vi "ABB Run Up report.vi"(10 "Report in":string) -> (2 "Report out":string)   [LabVIEW 2017]
uses:
  ABB global.vi
panel:
  out "Run Up Speed":T1(graph)
  out "Run Up Current":T1(graph)
  out "Run Up Voltage":T1(graph)
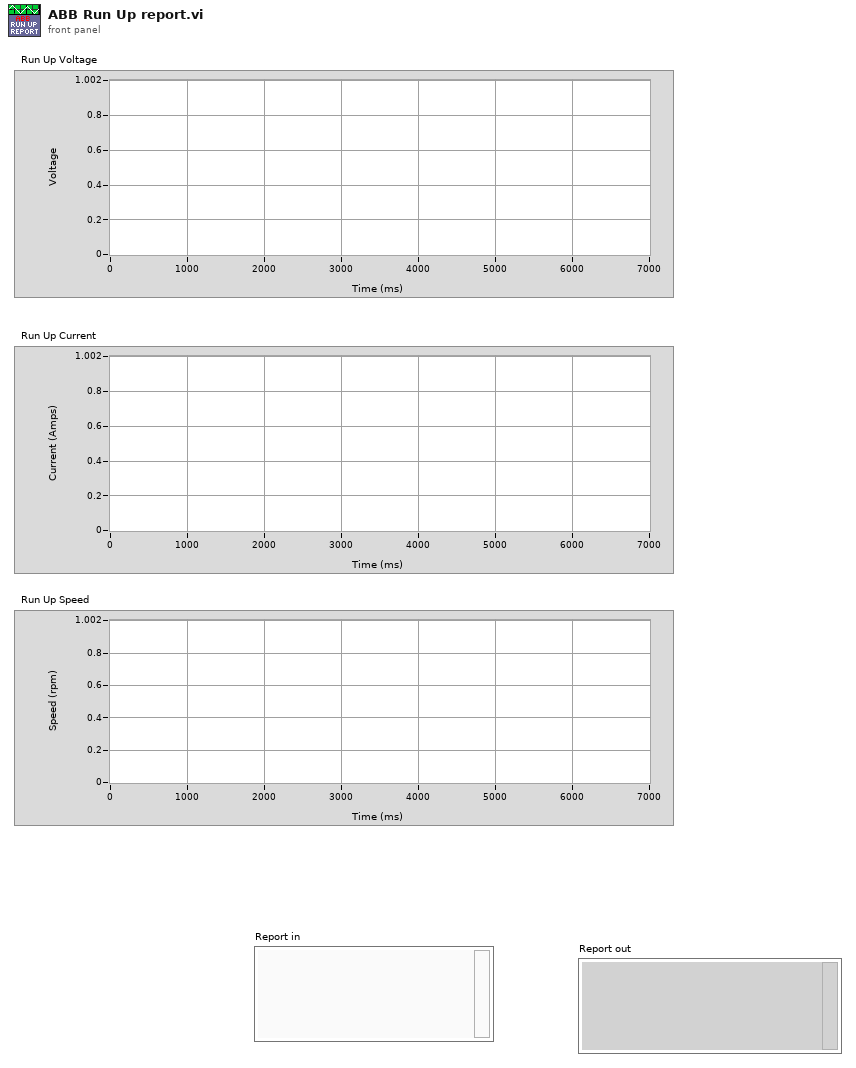
[diagram p1: front panel]
types:
  T1 = cluster{"No load test results":dbl[], "No load test results":dbl[]}
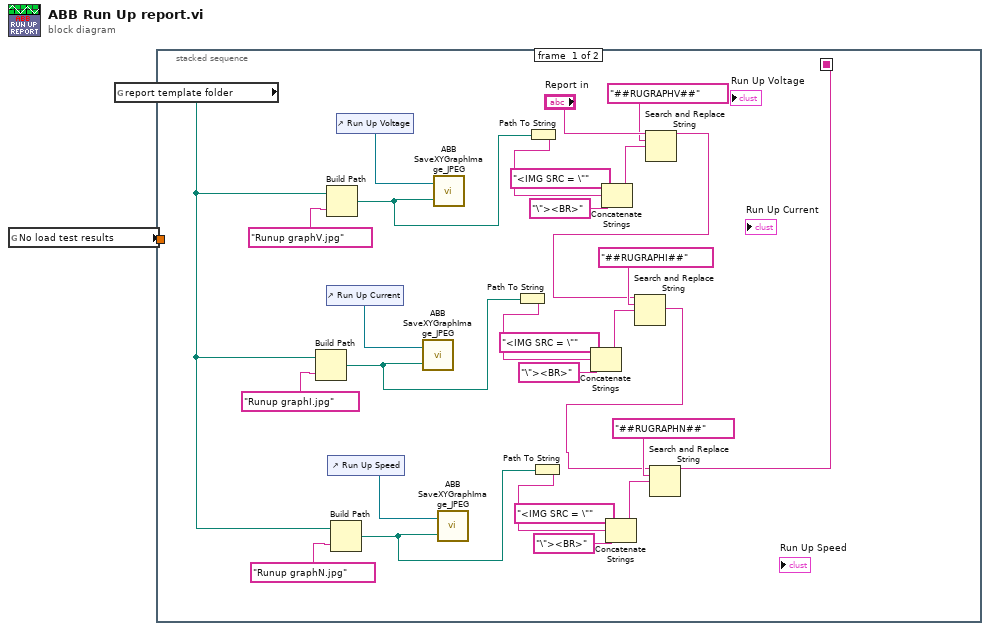
[diagram p0: block diagram]
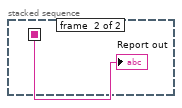
[diagram p2: hidden frame]
diagram:
  n1 = global read "ABB global.vi" "No load test results"() -> (w1:dbl[][])
  n2 = stacked-sequence {
    seq-local: [w2 _] -> [_ w31]
    tunnel: w1 -> [_ _]
    frame #0 {
      n3 = global read "ABB global.vi" "report template folder"() -> (w7:path)
      n4 = Build Path(base path=w7, name or relative path="Runup graphI.jpg") -> (appended path=w18:path)
      n5 = Build Path(base path=w7, name or relative path="Runup graphV.jpg") -> (appended path=w26:path)
      n6 = control-ref of="Run Up Current"() -> (w6:refnum<vi>)
      n7 = control-ref of="Run Up Speed"() -> (w5:refnum<vi>)
      n8 = Build Path(base path=w7, name or relative path="Runup graphN.jpg") -> (appended path=w11:path)
      n9 = control-ref of="Run Up Voltage"() -> (w30:refnum<vi>)
      n10 = call "ABB SaveXYGraphImage_JPEG.vi"("Path"=w18, "COntrolReference"=w6) -> ()  [unwired: 2 in]
      n11 = call "ABB SaveXYGraphImage_JPEG.vi"("Path"=w26, "COntrolReference"=w30) -> ()  [unwired: 2 in]
      n12 = call "ABB SaveXYGraphImage_JPEG.vi"("Path"=w11, "COntrolReference"=w5) -> ()  [unwired: 2 in]
      n13 = Path To String(path=w18) -> (string=w19:string)
      n14 = Path To String(path=w26) -> (string=w25:string)
      n15 = Path To String(path=w11) -> (string=w10:string)
      n16 = Concatenate Strings("<IMG SRC = \"", w19, "\"><BR>" ("string")) -> (w17:string)
      n17 = Concatenate Strings("<IMG SRC = \"", w25, "\"><BR>" ("string")) -> (w27:string)
      n18 = Concatenate Strings("<IMG SRC = \"", w10, "\"><BR>" ("string")) -> (w12:string)
      n19 = Search and Replace String(input string="Report in", search string="##RUGRAPHV##", replace string=w27) -> (result string=w4:string)  [unwired: 5 in, 3 out]
      n20 = Search and Replace String(input string=w4, search string="##RUGRAPHI##", replace string=w17) -> (result string=w3:string)  [unwired: 5 in, 3 out]
      n21 = Search and Replace String(input string=w3, search string="##RUGRAPHN##", replace string=w12) -> (result string=w2:string)  [unwired: 5 in, 3 out]
    }
    frame #1 {
      "Report out" <- w31
    }
  }
